vi "Module Type.vi"(11 "Event Viewer Module in":refnum<class "Event Viewer Module.lvclass">) -> (2 "Module Type":string)   [LabVIEW 2020, in "VolatusGUI.lvlib" / "Event Viewer Module.lvclass"]
uses:
  Event Viewer Module.lvclass
  Event Viewer Module.lvclass/Event Viewer Module.ctl
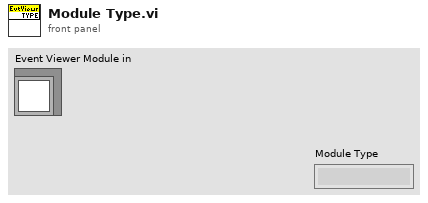
[diagram p1: front panel]
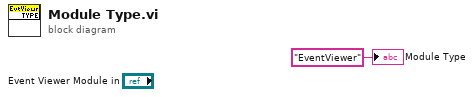
[diagram p0: block diagram]
diagram:
  "Module Type" <- "EventViewer" ("Module Type")
